vi "Pack Data.vi"(7 "Packed Offset In":i32, 8 "error in (no error)":errorcluster, 9 "Data Encoding":T1, 10 "CIPC Data":u8[](array[numeric]) format="%.0x", 11 "Packed Data In":u8[](array[numeric]) format="%.0x") -> (0 "error out":errorcluster, 3 "Packed Data Out":u8[](array[numeric]) format="%.0x", 5 "Packed Offset Out":i32)   [LabVIEW 2021, in "CIF_NI_CIPC.lvlib"]
doc: "Pack the encoded CIPC data to reduce size."
uses:
  CIF_NI_CIPC.lvlib
  TypeDefs/Data Encoding.ctl
  TypeDefs/Alignment.ctl
  <vilib>/CIF Foundation/CIF Utilities/DataTypes/Typedef/Endian.ctl
  TypeDefs/Data Struct Array Info.ctl
  TypeDefs/Data Element.ctl
  <vilib>/Utility/Data Type/Type Definitions/Data Type.ctl
  TypeDefs/Errors.ctl
  <vilib>/CIF Foundation/CIF Utilities/Errors/Append Error Location.vi
  <vilib>/CIF Foundation/CIF Utilities/DataTypes/DataTypes_CIF_U.lvlib
  <vilib>/Utility/Data Type/NI_Data Type.lvlib
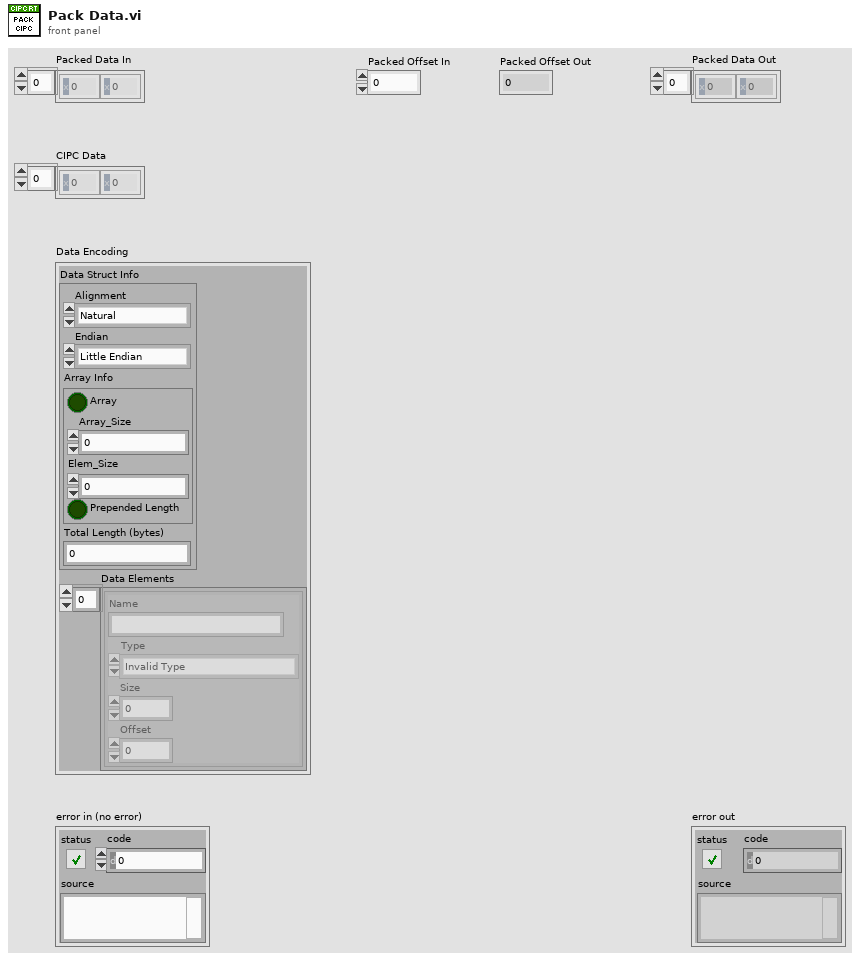
[diagram p1: front panel]
types:
  T1 = typedef "CIF_NI_CIPC.lvlib/Data Encoding.ctl" = cluster{"Data Struct Info":cluster{"Alignment":T2, "Endian":T3, "Array Info":T4, "Total Length (bytes)":i32}, "Data Elements":T5[]}
  T2 = typedef "CIF_NI_CIPC.lvlib/Alignment.ctl" = enum16{"Natural", "Packed"}
  T3 = typedef "DataTypes_CIF_U.lvlib/Endian.ctl" = enum16{"Little Endian", "Big Endian"}
  T4 = typedef "CIF_NI_CIPC.lvlib/Data Struct Array Info.ctl" = cluster{"Array":bool, "Array_Size":i32, "Elem_Size":i32, "Prepended Length":bool}
  T5 = typedef "CIF_NI_CIPC.lvlib/Data Element.ctl" = cluster{"Name":string, "Type":T6, "Size":u32, "Offset":u32}
  T6 = typedef "NI_Data Type.lvlib/Data Type.ctl" = enum8{"Invalid Type", "Void", "I8", "I16", "I32", "I64", "U8", "U16", "U32", "U64", "Single Float", "Double Float", "Extended Float", "Single Complex", "Double Complex", "Extended Complex", "Enum U8", "Enum U16", "Enum U32", "Enum U64", "Single Float With Unit", "Double Float With Unit", "Extended Float With Unit", "Single Complex with Unit", "Double Complex with Unit", "Extended Complex with Unit", "Boolean", "String", "Path", "Picture", "Tag", "Array", "Cluster", "Variant", "LV Variant", "Waveform", "Timestamp", "Digital Waveform", "Digital Data", "ExpressData", "Refnum", "External Data", "VI", "Poly VI", "LabVIEW Class Instance", "Fixed Point", "Set Collection", "Map Collection"}
  T7 = typedef "CIF_NI_CIPC.lvlib/Errors.ctl" = enum16{"Invalid Pack Length", "Invalid Pack Destination", "Unsupported Type", "Missing Library"}
  T8 = cluster{"Alignment":T2, "Endian":T3, "Array Info":T4, "Total Length (bytes)":i32}
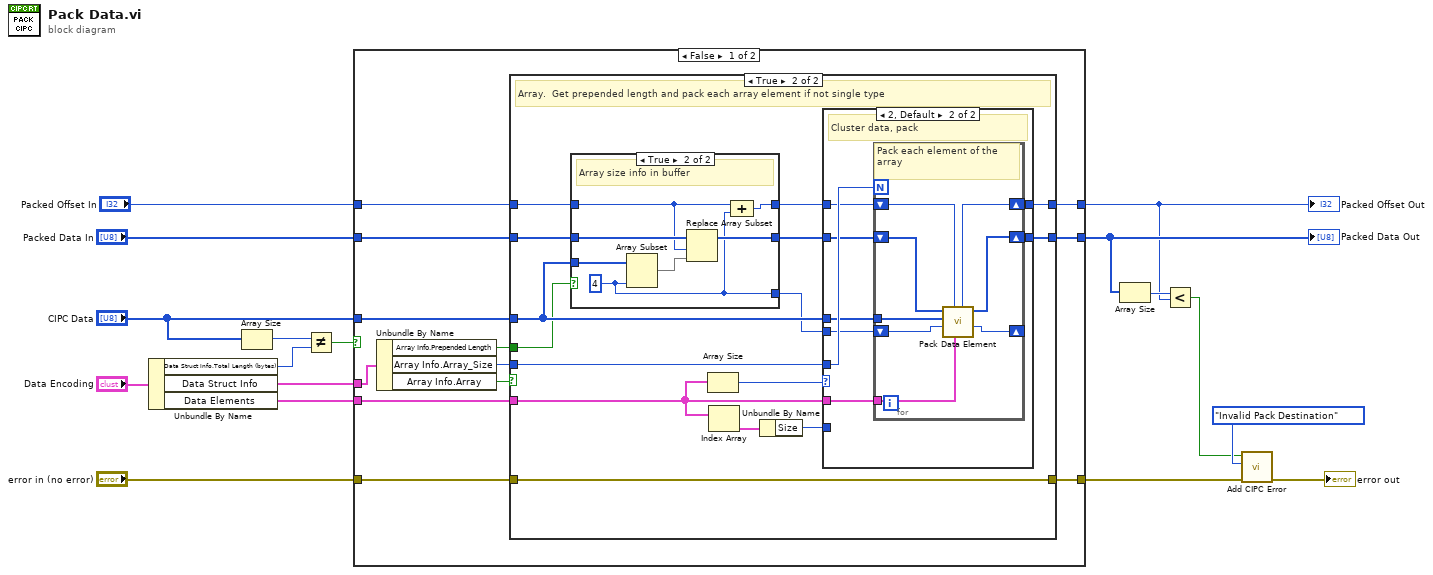
[diagram p0: block diagram]
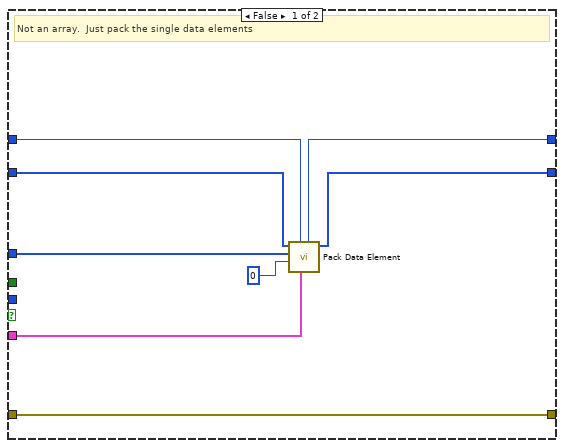
[diagram p2: hidden frame]
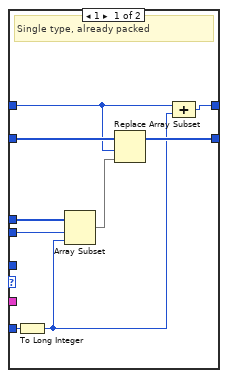
[diagram p3: hidden frame]
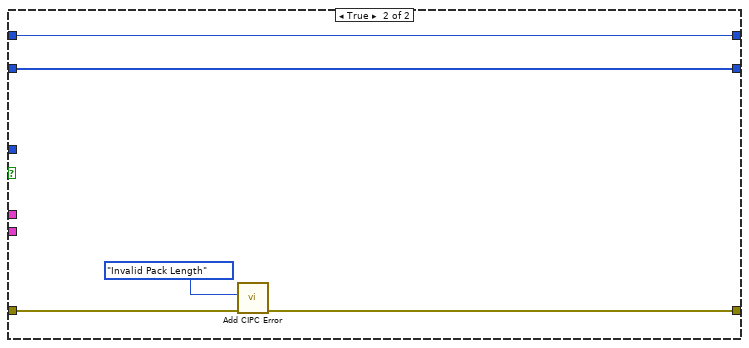
[diagram p5: hidden frame]
diagram:
  n1 = Unbundle By Name("Data Encoding") -> ("Data Struct Info.Total Length (bytes)"=w16:i32, "Data Struct Info"=w11:T8, "Data Elements"=w10:T5[])
  n2 = Array Size(array="CIPC Data") -> (size(s)=w15:i32)
  n3 = Not Equal?(x=w15, y=w16) -> (x != y?=w13:bool)
  n4 = case shown="False" w13 {
    tunnel: "error in (no error)" -> [w20 w91]
    tunnel: [w21 w90] -> w2
    tunnel: "CIPC Data" -> [w25 _]
    tunnel: w11 -> [w29 _]
    tunnel: w10 -> [w24 _]
    tunnel: "Packed Data In" -> [w23 w88]
    tunnel: [w22 w88] -> w7
    tunnel: "Packed Offset In" -> [w19 w87]
    tunnel: [w18 w87] -> w5
    frame False {
      n5 = Unbundle By Name(w29) -> ("Array Info.Prepended Length"=w26:bool, "Array Info.Array_Size"=w27:i32, "Array Info.Array"=w28:bool)
      n6 = case shown="True" w28 {
        tunnel: w27 -> [_ w52]
        tunnel: w26 -> [_ w44]
        tunnel: w25 -> [w31 w45]
        tunnel: w24 -> [w34 w41]
        tunnel: w23 -> [w37 w49]
        tunnel: [w36 w50] -> w22
        tunnel: [w35 w38] -> w21
        tunnel: w20 -> [w35 w38]
        tunnel: w19 -> [w33 w47]
        tunnel: [w32 w51] -> w18
        frame False {
          # "Not an array.  Just pack the single data elements"
          n7 = call "Pack Data Element.vi"("Data Elements"=w34, "Packed Offset In"=w33, "CIPC Offset In"=0, "CIPC Data"=w31, "Packed Data In in"=w37) -> ("Packed Data In out"=w36:u8[], "Packed Offset Out"=w32:i32)  [unwired: 4 in, 1 out]
        }
        frame True {
          # "Array.  Get prepended length and pack each array element if not single type"
          n8 = case shown="True" w44 {
            tunnel: w49 -> [w79 w86]
            tunnel: [w79 w85] -> w48
            tunnel: w47 -> [w78 w81]
            tunnel: [w78 w84] -> w46
            tunnel: w45 -> [_ w82]
            tunnel: [_ w80] -> w43
            frame False {
              # "No array size added"
            }
            frame True {
              w80 = 4 ("value")
              # "Array size info in buffer"
              n9 = Array Subset(array=w82, length=w80) -> (w83:u8[])  [unwired: 1 in]
              n10 = Replace Array Subset(array=w86, new element=w83, index=w81) -> (w85:u8[])
              n11 = Compound Arithmetic op=ADD(w81, w80) -> (w84:i32)
            }
          }
          n12 = Array Size(array=w41) -> (size(s)=w42:i32)
          n13 = Index Array(array=w41) -> (element=w40:T5)  [unwired: 1 in]
          n14 = Unbundle By Name(w40) -> ("Size"=w39:u32)
          n15 = case shown="2, Default" w42 {
            tunnel: w52 -> [_ w69]
            tunnel: [w59 w68] -> w51
            tunnel: [w60 w67] -> w50
            tunnel: w48 -> [w61 w66]
            tunnel: w46 -> [w54 w65]
            tunnel: w45 -> [w58 w64]
            tunnel: w43 -> [w55 w63]
            tunnel: w41 -> [_ w62]
            tunnel: w39 -> [w56 _]
            frame 1 {
              # "Single type, already packed"
              n16 = To Long Integer(number=w56) -> (32bit integer=w53:i32)
              n17 = Array Subset(array=w58, index=w55, length=w53) -> (w57:u8[])
              n18 = Replace Array Subset(array=w61, new element=w57, index=w54) -> (w60:u8[])
              n19 = Compound Arithmetic op=ADD(w54, w53) -> (w59:i32)
            }
            frame 2, Default {
              # "Cluster data, pack"
              n20 = for {
                N: w69 -> [_]
                tunnel: w62 -> [w76]
                tunnel: w64 -> [w75]
                shift-right: [w73] -> w67
                shift-left: w66 -> [w74]
                shift-right: [w72] -> w68
                shift-left: w65 -> [w77]
                shift-right: [w70] -> _
                shift-left: w63 -> [w71]
                # "Pack each element of the array"
                n21 = call "Pack Data Element.vi"("Data Elements"=w76, "Packed Offset In"=w77, "CIPC Offset In"=w71, "CIPC Data"=w75, "Packed Data In in"=w74) -> ("CIPC Offset Out"=w70:i32, "Packed Data In out"=w73:u8[], "Packed Offset Out"=w72:i32)  [unwired: 4 in]
              }
            }
          }
        }
      }
    }
    frame True {
      n22 = call "Add CIPC Error.vi"("error in (no error)"=w91, "Error"=Errors."Invalid Pack Length") -> ("error out"=w90:errorcluster)  [unwired: 9 in]
    }
  }
  "Packed Data Out" <- w7
  "Packed Offset Out" <- w5
  n23 = Array Size(array=w7) -> (size(s)=w6:i32)
  n24 = Less?(x=w6, y=w5) -> (x < y?=w3:bool)
  n25 = call "Add CIPC Error.vi"("error in (no error)"=w2, "Error"=Errors."Invalid Pack Destination", "Insert Error"=w3) -> ("error out"=→"error out":errorcluster)  [unwired: 8 in]
